vi "Enter User String.vi"(8 "error in (no error)":errorcluster, 9 "Caption":string, 10 "Clear Value (F)":bool, 11 "Message":string="Please enter the beta code to unlock beta features:") -> (0 "error out":errorcluster, 1 "OK":bool, 3 "User entered string":string caption="Code")   [LabVIEW 2021, in "Strings.lvlib"]
doc: "Displays a standard dialog box that prompts users to enter information, such as a user name and password.\n--------------------\n\nThis Express VI is configured as follows:\n\nMessage to Display to the User:Please enter the beta code to unlock beta features:\nThe inputs are: \nText Entry Box: Code"
uses:
  Strings/Strings.lvlib
panel:
  in  "Code":string
  out "String":string="Please enter the beta code to unlock beta features:"
  in  "OK1":bool
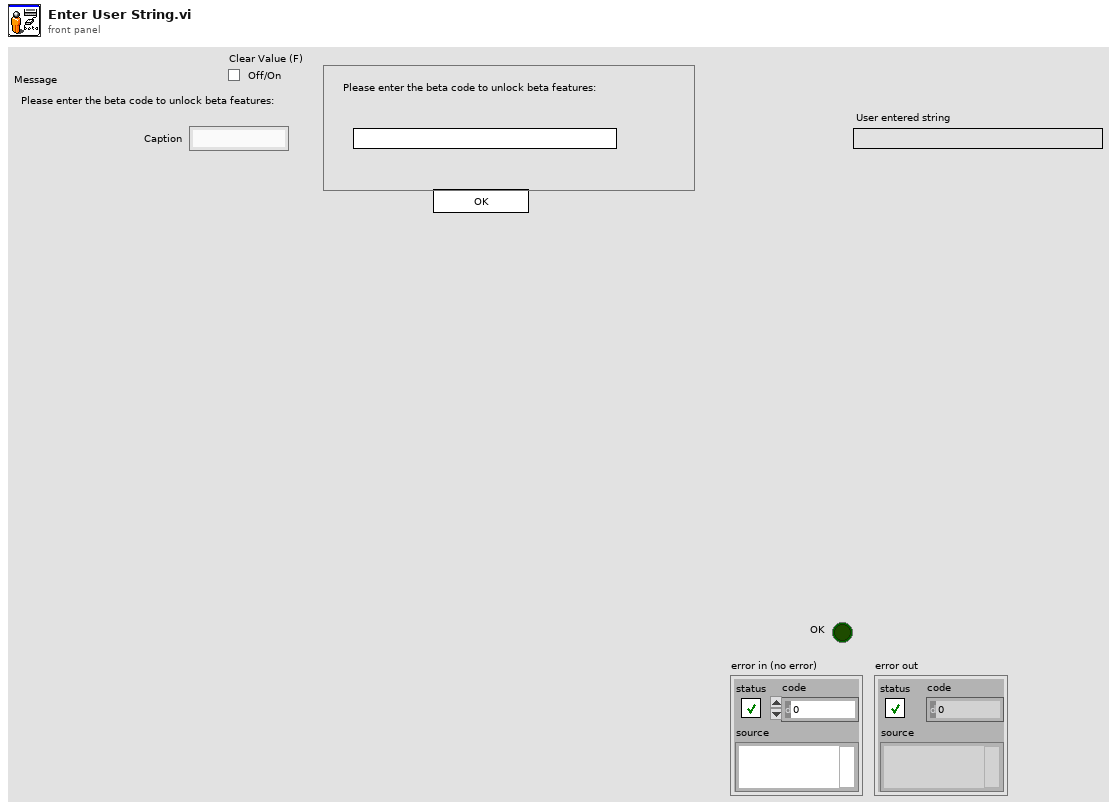
[diagram p1: front panel]
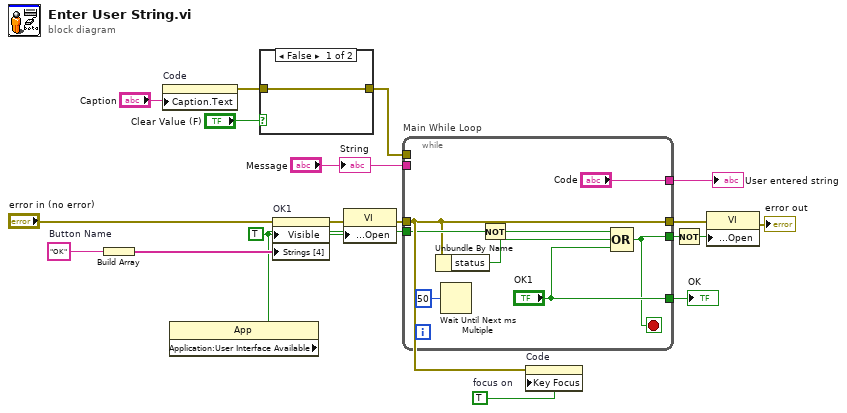
[diagram p0: block diagram]
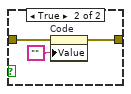
[diagram p2: hidden frame]
diagram:
  w9 = TRUE  # focus on
  w15 = "OK"  # Button Name
  n1 = Build Array(w15) -> (w16:string[])
  n2 = property on="Code" class="Str"("Caption.Text"="Caption") -> (error out=w3:errorcluster)  [unwired: 2 in, 1 out]
  n3 = property class="App"() -> ("Application:User Interface Available"=w6:bool)  [unwired: 2 in, 2 out]
  n4 = case shown="False" "Clear Value (F)" {
    tunnel: w3 -> [w20 w23]
    tunnel: [w20 w22] -> w2
    frame False {
    }
    frame True {
      n5 = property on="Code" class="Str"(error in=w23, "Value"="") -> (error out=w22:errorcluster)  [unwired: 1 in, 1 out]
    }
  }
  n6 = property on="OK1" class="Bool"(error in="error in (no error)", "Visible"=TRUE, "Strings [4]"=w16) -> (error out=w14:errorcluster)  [unwired: 1 in, 1 out]
  n7 = property class="VI"(error in=w14, "Front Panel Window:Open"=w6) -> (error out=w13:errorcluster)  [unwired: 1 in, 1 out]
  n8 = while "Main While Loop" {
    tunnel: ["OK1"] -> w19
    tunnel: w6 -> [w29]
    tunnel: [w27] -> w17
    tunnel: w13 -> [w26]
    tunnel: [w26] -> w12
    tunnel: ["Code"] -> w10
    tunnel: w2 -> [_]
    tunnel: "Message" -> [_]
    stop <- w27 stop-if-true
    n9 = Unbundle By Name(w26) -> ("status"=w25:bool)
    n10 = Wait Until Next ms Multiple(millisecond multiple=u32 50) -> ()  [unwired: 1 out]
    n11 = Not(x=w29) -> (.not. x?=w28:bool)
    n12 = Compound Arithmetic op=OR(w28, w25, "OK1") -> (w27:bool)
  }
  "OK" <- w19
  "User entered string" <- w10
  n13 = property on="Code" class="Str"(error in=w13, "Key Focus"=w9) -> ()  [unwired: 1 in, 2 out]
  n14 = Not(x=w17) -> (.not. x?=w18:bool)
  n15 = property class="VI"(error in=w12, "Front Panel Window:Open"=w18) -> (error out=→"error out":errorcluster)  [unwired: 1 in, 1 out]
  "String" <- "Message"
